vi "Main.vi"(8 "error in (no error)":errorcluster, 11 "GalvoBase in":refnum<class "ImagingModeSPIM.lvclass">) -> (0 "error out":errorcluster, 3 "component":refnum<class "ImagingModeSPIM.lvclass">)   [LabVIEW 2012, in "ImagingModeSPIM.lvclass"]
doc: "Main VI of the component."
uses:
  ImagingModeSPIM.lvclass
  Controls/wavelength_ring.ctl
  ImagingModeSPIM.lvclass/ImagingModeSPIM.ctl
  <vilib>/Distrio/Murmex/InitialiseMessage/InitialiseMessage.lvclass
  <vilib>/Distrio/Murmex/TerminateMessage/TerminateMessage.lvclass
  <vilib>/Distrio/Murmex/ConfigureMessage/ConfigureMessage.lvclass
  <vilib>/Distrio/Murmex/StopMessage/StopMessage.lvclass
  <vilib>/Distrio/Murmex/StartMessage/run mode enum.ctl
  <vilib>/Distrio/Murmex/StartMessage/StartMessage.lvclass
  <vilib>/Distrio/Murmex/Murmex/update_cluster.ctl
  <vilib>/Distrio/Murmex/Murmex/Set configure at initialise.vi
  <vilib>/Distrio/Murmex/Murmex/Set VI reference.vi
  <vilib>/Distrio/Murmex/Murmex/Get ID.vi
  <vilib>/Distrio/Murmex/Murmex/Set relay start stop to observers.vi
  <vilib>/Distrio/Murmex/Murmex/Set log reference.vi
  <vilib>/Distrio/Murmex/Murmex/Set license required.vi
  <vilib>/Distrio/Murmex/Murmex/Set write log to disk.vi
  <vilib>/Distrio/Murmex/StartMessage/Set run mode.vi
  <vilib>/Distrio/Murmex/Murmex/Murmex.lvclass
panel:
  in  "button::quit":bool
  in  "button:start_finite":bool
  in  "button:start_free-run":bool
  in  "button::configure":bool
  in  "Tab Control":T1(tab)
  in  "Phase 2":dbl[unit] caption="phase" min=-6.283185307179586 max=6.283185307179586 step=0.0017453292519943296
  in  "Offset 2":dbl[unit] caption="offset" min=-5.0 max=5.0 step=0.01
  in  "Amplitude 2":dbl[unit]=1.0 caption="amplitude" min=0.0 max=5.0 step=0.01
  in  "Phase 1":dbl[unit] caption="phase" min=-6.283185307179586 max=6.283185307179586 step=0.0017453292519943296
  in  "Offset 1":dbl[unit] caption="offset" min=-5.0 max=5.0 step=0.01
  in  "Amplitude 1":dbl[unit]=1.0 caption="amplitude" min=0.0 max=5.0 step=0.01
  out "Offset_slow":dbl[unit] caption="offset"
  out "step_size":dbl[unit]=1.0 caption="step size"
  in  "Phase_fast":dbl[unit]=3.141593 caption="phase" min=-6.283185307179586 max=6.283185307179586 step=0.0017453292519943296
  in  "Offset_fast":dbl[unit] caption="offset" min=-5.0 max=5.0 step=0.01
  in  "Amplitude_fast":dbl[unit]=0.5 caption="amplitude" min=-10.0 max=10.0 step=0.01
  out "write to task counter":i32
  out "data sent":dbl[unit]
  out "frequency slow":dbl[unit]
  in  "additional offset":dbl[unit]
  out "frame rate":dbl[unit]=100.0
  out "HSYNC pulses":i32=2048 min=4 max=2048 step=4
  in  "Wavelength":T2 items=["405nm"=0.14, "445nm"=0.34, "491nm"=0.41, "515nm"=0.17, "561nm"=0.5]
  in  "digital ratio":dbl(knob)=0.5 min=0.0 max=1.0 step=0.02 scale=0.0..1.0
  in  "pulses per pixel":i32=2 min=0 max=20 step=2
  out "log":string
  in  "ID":string="spim"
  out "terminate?":bool=TRUE
  # "galvo 1"
  # "galvo 2"
  # "fast scan"
  # "slow scan"
  # "Prato"
  # "Florence"
  # "ImagingModeSPIM\n\nDeveloped by:\n\nMarcel van 't Hoff PhD, \nMarie Caroline Muellenbroich PhD, \nLudovico Silvestri PhD,\nUniversity of Florence, 2014"
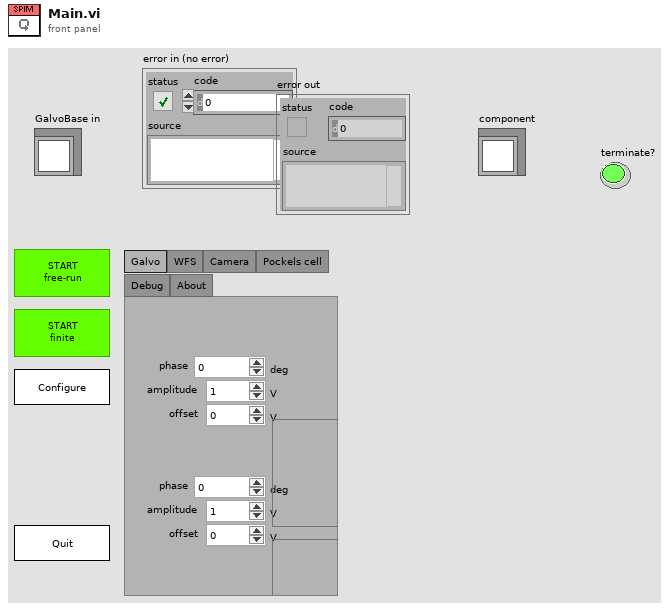
[diagram p1: front panel]
types:
  T1 = enum32{"Galvo", "WFS", "Camera", "Pockels cell", "Debug", "About"}
  T2 = typedef "ImagingModeSPIM.lvclass/wavelength_ring.ctl" = dbl
  T3 = enum8{"Enabled", "Disabled", "Disabled and Grayed Out"}
  T4 = typedef "Murmex.lvlib/StartMessage.lvclass/run mode enum.ctl" = enum16{"infinite", "finite"}
  T5 = typedef "Murmex.lvlib/Murmex.lvclass/update_cluster.ctl" = cluster{"target ID":string, "key chains":string[], "values":variant[]}
  T6 = typedef "Murmex.lvlib/Murmex.lvclass/command_enum.ctl" = enum16{"null", "initialise", "reset", "terminate", "acknowledge", "update", "inspect", "inform", "proceed", "start", "stop", "fetch", "configure", "generic"}
  T7 = typedef "Murmex.lvlib/Murmex.lvclass/Event type enumerations.ctl" = enum16{"before", "after"}
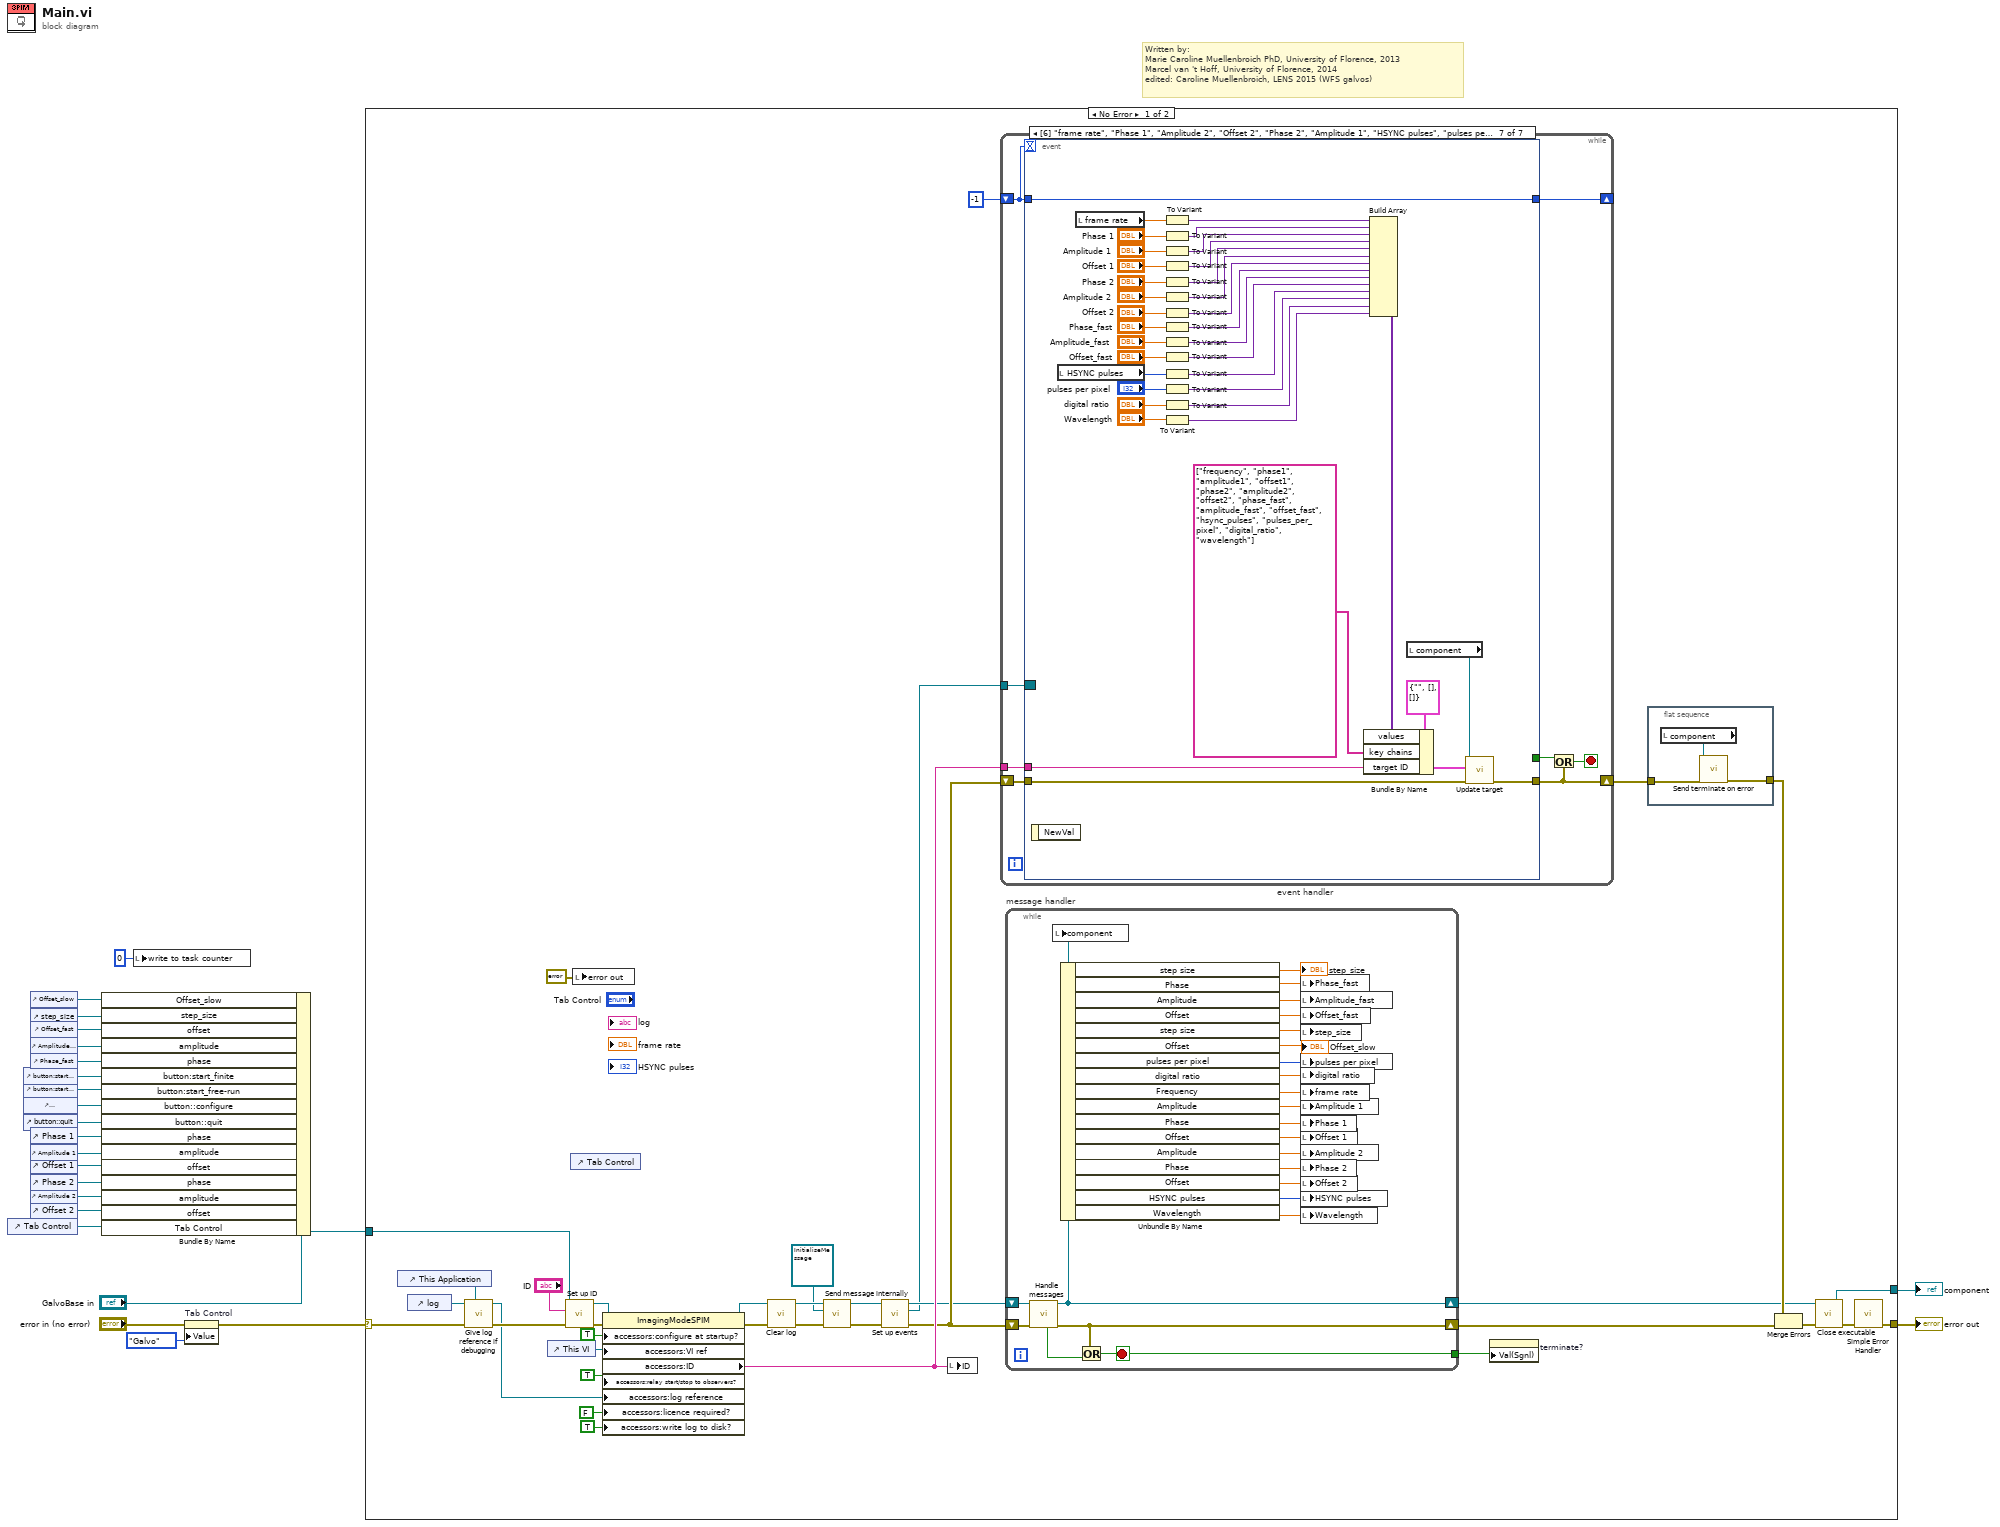
[diagram p0: block diagram]
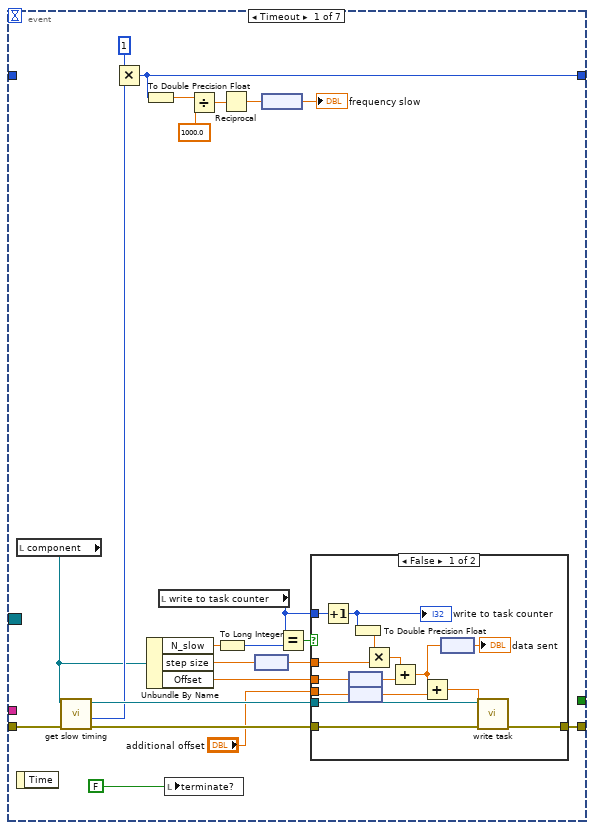
[diagram p2: hidden frame]
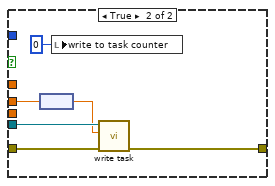
[diagram p3: hidden frame]
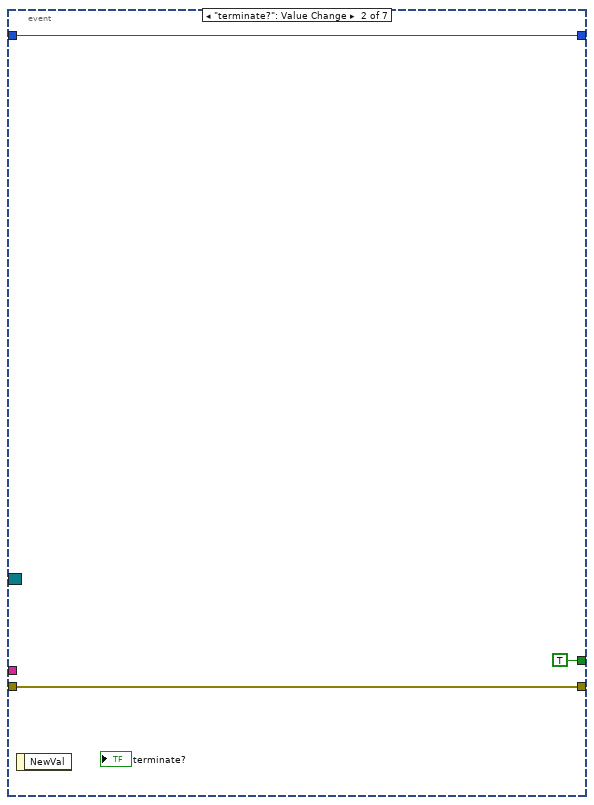
[diagram p4: hidden frame]
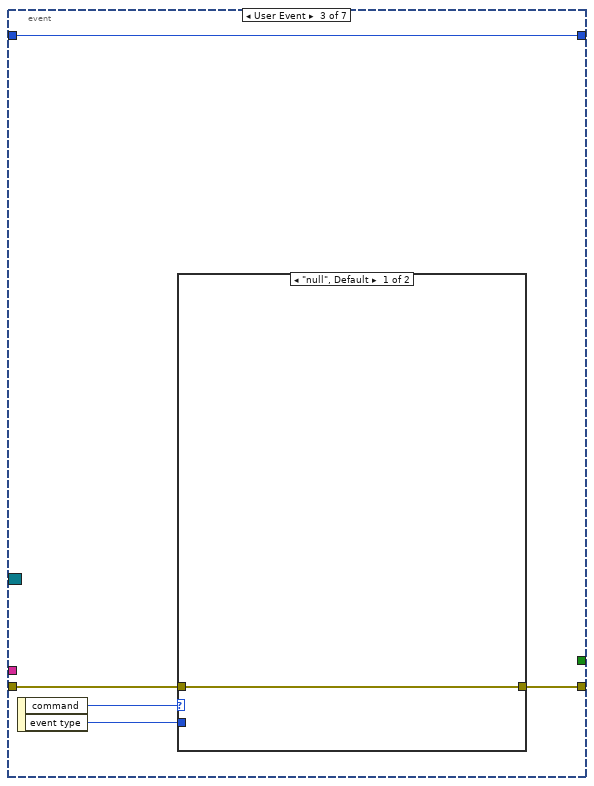
[diagram p5: hidden frame]
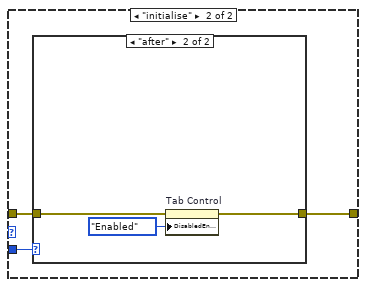
[diagram p6: hidden frame]
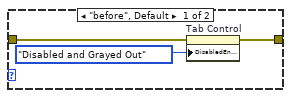
[diagram p7: hidden frame]
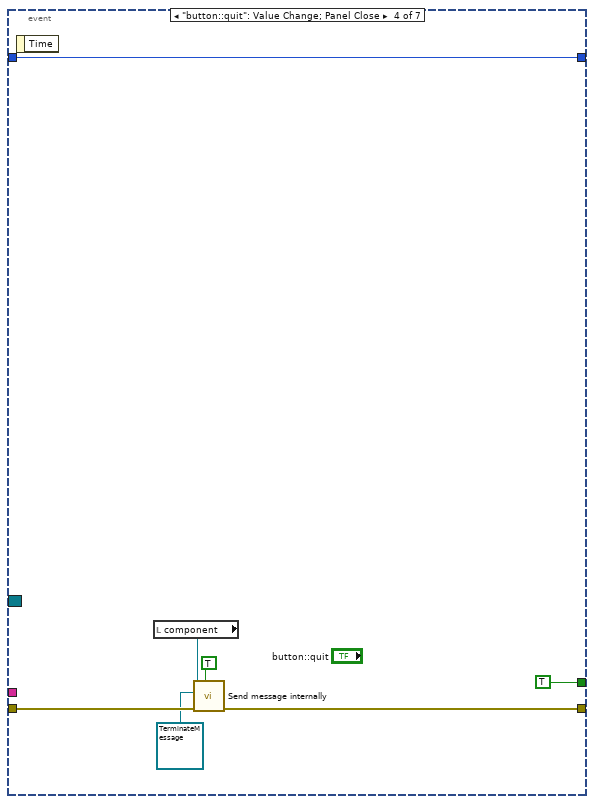
[diagram p8: hidden frame]
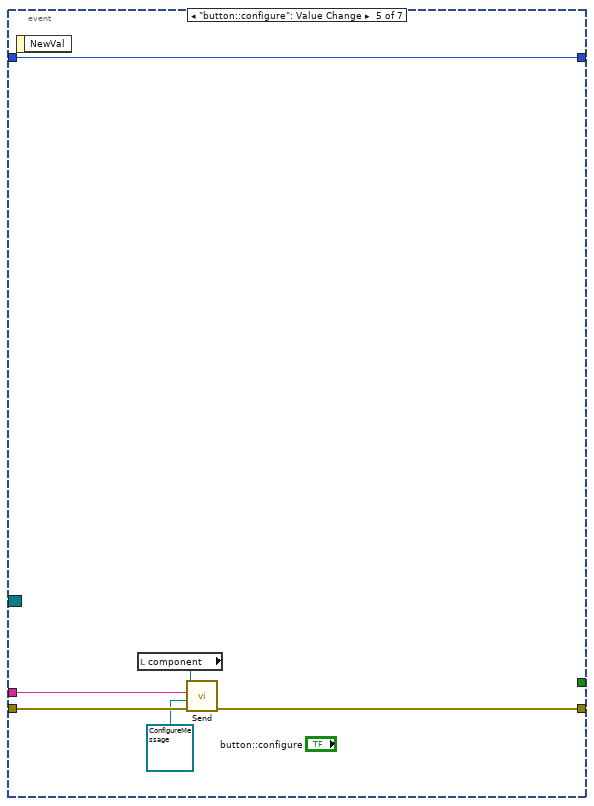
[diagram p9: hidden frame]
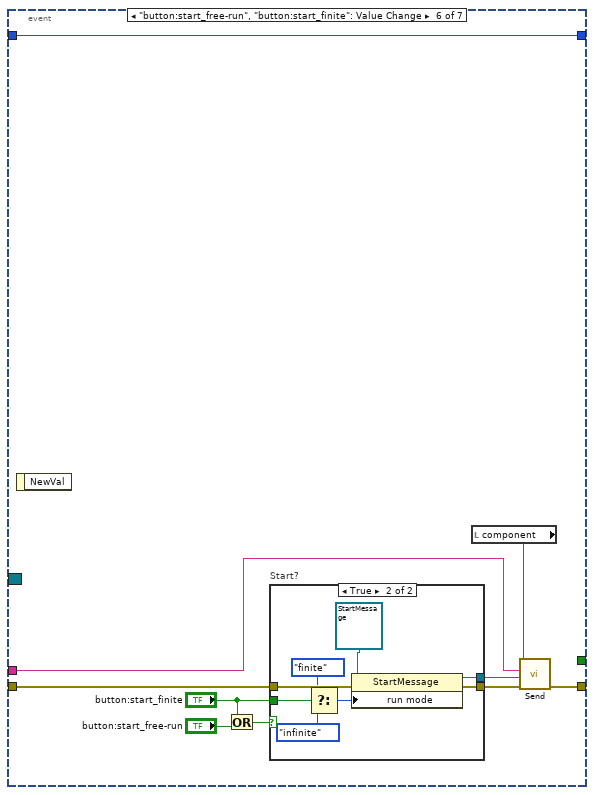
[diagram p10: hidden frame]
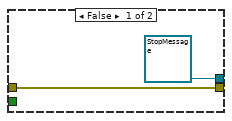
[diagram p11: hidden frame]
diagram:
  # "Written by:\nMarie Caroline Muellenbroich PhD, University of Florence, 2013 \nMarcel van 't Hoff, University of Florence, 2014\nedited: Caroline Muellenbroich, LENS 2015 (WFS galvos)"
  n1 = control-ref of="Tab Control"() -> (w4:refnum<vi>)
  n2 = control-ref of="button:start_finite"() -> (w21:refnum<vi>)
  n3 = control-ref of="button:start_free-run"() -> (w18:refnum<vi>)
  n4 = control-ref of="button::configure"() -> (w19:refnum<vi>)
  n5 = control-ref of="button::quit"() -> (w20:refnum<vi>)
  n6 = control-ref of="Offset_slow"() -> (w3:refnum<vi>)
  n7 = control-ref of="step_size"() -> (w2:refnum<vi>)
  n8 = control-ref of="Offset_fast"() -> (w6:refnum<vi>)
  n9 = control-ref of="Amplitude_fast"() -> (w7:refnum<vi>)
  n10 = control-ref of="Phase_fast"() -> (w8:refnum<vi>)
  n11 = control-ref of="Phase 1"() -> (w17:refnum<vi>)
  n12 = control-ref of="Amplitude 1"() -> (w16:refnum<vi>)
  n13 = control-ref of="Offset 1"() -> (w15:refnum<vi>)
  n14 = control-ref of="Phase 2"() -> (w14:refnum<vi>)
  n15 = control-ref of="Amplitude 2"() -> (w13:refnum<vi>)
  n16 = control-ref of="Offset 2"() -> (w12:refnum<vi>)
  n17 = Bundle By Name(cluster="GalvoBase in", "Offset_slow"=w3, "step_size"=w2, "offset"=w6, "amplitude"=w7, "phase"=w8, "button:start_finite"=w21, "button:start_free-run"=w18, "button::configure"=w19, "button::quit"=w20, "phase"=w17, "amplitude"=w16, "offset"=w15, "phase"=w14, "amplitude"=w13, "offset"=w12, "Tab Control"=w4) -> (w22:refnum<class "ImagingModeSPIM.lvclass">)
  n18 = local write "write to task counter"(0 ("write to task counter")) -> ()
  n19 = property on="Tab Control" class="TabCtl (strict)"(error in="error in (no error)", "Value"=T1."Galvo" ("Tab Control")) -> (error out=w9:errorcluster)  [unwired: 1 in, 1 out]
  n20 = case shown="No Error" w9 {
    selector: w9 -> [w30 w226]
    tunnel: [w60 w226] -> w24
    tunnel: w22 -> [w42 w227]
    tunnel: [w59 w227] -> w10
    frame No Error {
      n21 = control-ref of="This Application"() -> (w26:refnum<vi>)
      n22 = control-ref of="log"() -> (w28:refnum<vi>)
      n23 = call "Give log reference if debugging.vi"("application ref"=w26, "error in (no error)"=w30, "log reference in"=w28) -> ("error out"=w29:errorcluster, "log reference out"=w27:refnum<vi>)  [unwired: 6 in, 1 out]
      n24 = control-ref of="This VI"() -> (w57:refnum<vi>)
      n25 = call <vilib>:"Set up ID.vi"("error in (no error)"=w29, "component ID"="ID", "MurmexBase in"=w42) -> ("error out"=w54:errorcluster, "MurmexBase out"=w55:refnum<class "ImagingModeSPIM.lvclass">)  [unwired: 6 in, 1 out]
      n26 = control-ref of="Tab Control"() -> ()  [unwired: 1 out]
      n27 = local write "error out"(errorcluster {"status"=FALSE, "code"=0, "source"=""} ("error out")) -> ()
      n28 = property class="ImagingModeSPIM"(reference=w55, error in=w54, "accessors:configure at startup?"=TRUE ("configure at startup?"), "accessors:VI ref"=w57, "accessors:relay start/stop to observers?"=TRUE ("relay start/stop to observers?"), "accessors:log reference"=w27, "accessors:licence required?"=FALSE ("licence required?"), "accessors:write log to disk?"=TRUE ("write log to disk?")) -> (reference out=w39:refnum<class "ImagingModeSPIM.lvclass">, error out=w41:errorcluster, "accessors:ID"=w44:string)
      n29 = call <vilib>:"Clear log.vi"("error in (no error)"=w41, "MurmexBase in"=w39) -> ("error out"=w40:errorcluster, "MurmexBase out"=w38:refnum<class "ImagingModeSPIM.lvclass">)  [unwired: 8 in]
      n30 = call <vilib>:"Send message internally.vi"("error in (no error)"=w40, "Message"=refnum<class "InitialiseMessage.lvclass"> refnum ("Murmex.lvlib:InitialiseMessage"), "Murmex in"=w38) -> ("error out"=w35:errorcluster, "Murmex out"=w33:refnum<class "ImagingModeSPIM.lvclass">)  [unwired: 7 in]
      n31 = call <vilib>:"Set up events.vi"("error in (no error)"=w35, "MurmexBase in"=w33) -> ("error out"=w34:errorcluster, "Event Registration Refnum"=w31:refnum<event-registration>, "MurmexBase out"=w32:refnum<class "ImagingModeSPIM.lvclass">)  [unwired: 7 in]
      n32 = local write "ID"(w44) -> ()
      n33 = while "event handler" {
        shift-right: [w69] -> w52
        shift-left: w34 -> [w71]
        shift-right: [w65] -> _
        shift-left: -1 -> [w66]
        tunnel: w44 -> [w67]
        tunnel: w31 -> [w64]
        stop <- w68 stop-if-true
        n34 = event shown="[6] \"frame rate\", \"Phase 1\", \"Amplitude 2\", \"Offset 2\", \"Phase 2\", \"Amplitude 1\", \"HSYNC pulses\", \"pulses per pixel\", \"digital ratio\", \"Wavelength\", \"Offset_slow\", \"step_size\", \"Phase_fast\", \"Offset_fast\", \"Amplitude_fast\", \"Offset 1\": Value Change" {
          selector: w64 -> [_ _ _ _ _ _ _]
          dyn-events: _ -> [_ _ _ _ _ _ _]
          timeout: w66 -> [_ _ _ _ _ _ _]
          tunnel: [w92 w117 w119 w139 w144 w149 w201] -> w69
          tunnel: w71 -> [w91 w117 w120 w138 w145 w154 w202]
          tunnel: [_ TRUE ("configure at startup?") _ TRUE ("configure at startup?") _ _ _] -> w70
          tunnel: w67 -> [_ _ _ _ w143 w146 w183]
          tunnel: w66 -> [_ w115 w118 w136 w142 w155 w189]
          tunnel: [w78 w115 w118 w136 w142 w155 w189] -> w65
          event Timeout {
            n35 = local read "component"() -> (w86:refnum<class "ImagingModeSPIM.lvclass">)
            n36 = event-data() -> ()  [unwired: 1 in, 1 out]
            n37 = call-dynamic "get slow timing.vi"("error in (no error)"=w91, "ImagingModeSPIM in"=w86) -> ("error out"=w90:errorcluster, "frame rate"=w87:i32, "ImagingModeSPIM out"=w89:refnum<class "ImagingModeSPIM.lvclass">)  [unwired: 6 in, 1 out]
            n38 = Multiply(x=1, y=w87) -> (x*y=w78:i32)
            n39 = To Double Precision Float(number=w78) -> (double precision float=w77:dbl)
            n40 = Unbundle By Name(w86) -> ("N_slow"=w85:dbl, "step size"=w74:dbl[unit], "Offset"=w80:dbl[unit])
            n41 = local read "write to task counter"() -> (w83:i32)
            n42 = local write "terminate?"(FALSE ("terminate?")) -> ()
            n43 = Divide(x=w77, y=1000.0) -> (x/y=w76:dbl)
            n44 = To Long Integer(number=w85) -> (32bit integer=w82:i32)
            n45 = Reciprocal(x=w76) -> (1/x=w75:dbl)
            n46 = node(w74) -> (w81:dbl)
            n47 = node(w75) -> (→"frequency slow":dbl[unit])
            n48 = Equal?(x=w83, y=w82) -> (x = y?=w84:bool)
            n49 = case shown="False" w84 {
              tunnel: [w107 w114] -> w92
              tunnel: w90 -> [w108 w113]
              tunnel: w89 -> [w106 w112]
              tunnel: w83 -> [w105 _]
              tunnel: w81 -> [w103 _]
              tunnel: w80 -> [w100 w109]
              tunnel: "additional offset" -> [w95 _]
              frame False {
                n50 = Increment(x=w105) -> (x+1=w102:i32)
                "write to task counter" <- w102
                n51 = node(w100) -> (w99:dbl)
                n52 = node(w95) -> (w94:dbl)
                n53 = To Double Precision Float(number=w102) -> (double precision float=w104:dbl)
                n54 = Multiply(x=w104, y=w103) -> (x*y=w101:dbl)
                n55 = Add(x=w101, y=w99) -> (x+y=w98:dbl)
                n56 = Add(x=w98, y=w94) -> (x+y=w96:dbl)
                n57 = node(w98) -> (→"data sent":dbl[unit])
                n58 = call-dynamic "write task.vi"("error in (no error)"=w108, "data"=w96, "ImagingModeSPIM in"=w106) -> ("error out"=w107:errorcluster)  [unwired: 7 in, 1 out]
              }
              frame True {
                n59 = node(w109) -> (w110:dbl)
                n60 = local write "write to task counter"(0 ("write to task counter")) -> ()
                n61 = call-dynamic "write task.vi"("error in (no error)"=w113, "data"=w110, "ImagingModeSPIM in"=w112) -> ("error out"=w114:errorcluster)  [unwired: 7 in, 1 out]
              }
            }
          }
          event "terminate?": Value Change {
            n62 = event-data() -> ()  [unwired: 1 in, 1 out]
          }
          event User Event {
            n63 = event-data() -> ("command"=w122:T6, "event type"=w121:T7)  [unwired: 1 in]
            n64 = case shown="\"null\", Default" w122 {
              tunnel: w121 -> [_ w126]
              tunnel: w120 -> [w123 w125]
              tunnel: [w123 w124] -> w119
              frame "null", Default {
              }
              frame "initialise" {
                n65 = case shown="\"after\"" w126 {
                  tunnel: w125 -> [w129 w132]
                  tunnel: [w128 w131] -> w124
                  frame "before", Default {
                    n66 = property on="Tab Control" class="TabCtl (strict)"(error in=w129, "DisabledEnum"=T3."Disabled and Grayed Out" ("Disabled")) -> (error out=w128:errorcluster)  [unwired: 1 in, 1 out]
                  }
                  frame "after" {
                    n67 = property on="Tab Control" class="TabCtl (strict)"(error in=w132, "DisabledEnum"=T3."Enabled" ("Disabled")) -> (error out=w131:errorcluster)  [unwired: 1 in, 1 out]
                  }
                }
              }
            }
          }
          event "button::quit": Value Change; Panel Close {
            n68 = event-data() -> ()  [unwired: 1 in, 1 out]
            n69 = local read "component"() -> (w135:refnum<class "ImagingModeSPIM.lvclass">)
            n70 = call <vilib>:"Send message internally.vi"("priority message? (F)"=TRUE, "error in (no error)"=w138, "Message"=refnum<class "TerminateMessage.lvclass"> refnum ("Murmex.lvlib:TerminateMessage"), "Murmex in"=w135) -> ("error out"=w139:errorcluster)  [unwired: 6 in, 1 out]
          }
          event "button::configure": Value Change {
            n71 = event-data() -> ()  [unwired: 1 in, 1 out]
            n72 = local read "component"() -> (w141:refnum<class "ImagingModeSPIM.lvclass">)
            n73 = call <vilib>:"Send.vi"("error in (no error)"=w145, "Message"=refnum<class "ConfigureMessage.lvclass"> refnum ("Murmex.lvlib:ConfigureMessage"), "recipient"=w143, "Murmex in"=w141) -> ("error out"=w144:errorcluster)  [unwired: 6 in, 1 out]
          }
          event "button:start_free-run", "button:start_finite": Value Change {
            n74 = event-data() -> ()  [unwired: 1 in, 1 out]
            n75 = Or(x="button:start_finite", y="button:start_free-run") -> (x .or. y?=w153:bool)
            n76 = case "Start?" shown="True" w153 {
              tunnel: w154 -> [w157 w165]
              tunnel: [w157 w160] -> w150
              tunnel: "button:start_finite" -> [_ w161]
              tunnel: [refnum<class "StopMessage.lvclass"> refnum ("Murmex.lvlib:StopMessage") w159] -> w147
              frame False {
              }
              frame True {
                n77 = Select(t=run_mode_enum."finite" ("run mode"), s=w161, f=run_mode_enum."infinite" ("run mode")) -> (s? t:f=w162:T4)
                n78 = property class="StartMessage"(reference=refnum<class "StartMessage.lvclass"> refnum ("Murmex.lvlib:StartMessage"), error in=w165, "run mode"=w162) -> (reference out=w159:refnum<class "StartMessage.lvclass">, error out=w160:errorcluster)
              }
            }
            n79 = local read "component"() -> (w148:refnum<class "ImagingModeSPIM.lvclass">)
            n80 = call <vilib>:"Send.vi"("error in (no error)"=w150, "Message"=w147, "recipient"=w146, "Murmex in"=w148) -> ("error out"=w149:errorcluster)  [unwired: 6 in, 1 out]
          }
          event "frame rate", "Phase 1", "Amplitude 2", "Offset 2", "Phase 2", "Amplitude 1", "HSYNC pulses", "pulses per pixel", "digital ratio", "Offset_slow", "step_size", "Phase_fast", "Offset_fast", "Amplitude_fast", "Offset 1": Value Change {
            n81 = event-data() -> ()  [unwired: 1 in, 1 out]
            n82 = local read "HSYNC pulses"() -> (w180:i32)
            n83 = local read "frame rate"() -> (w179:dbl[unit])
            n84 = To Variant(anything=w179) -> (Variant=w198:variant)
            n85 = To Variant(anything="Phase 1") -> (Variant=w195:variant)
            n86 = To Variant(anything="Amplitude 1") -> (Variant=w194:variant)
            n87 = To Variant(anything="Offset 1") -> (Variant=w193:variant)
            n88 = To Variant(anything="Phase 2") -> (Variant=w187:variant)
            n89 = To Variant(anything="Amplitude 2") -> (Variant=w186:variant)
            n90 = To Variant(anything="Offset 2") -> (Variant=w184:variant)
            n91 = To Variant(anything="Phase_fast") -> (Variant=w173:variant)
            n92 = To Variant(anything="Amplitude_fast") -> (Variant=w172:variant)
            n93 = To Variant(anything="Offset_fast") -> (Variant=w171:variant)
            n94 = To Variant(anything=w180) -> (Variant=w170:variant)
            n95 = To Variant(anything="pulses per pixel") -> (Variant=w169:variant)
            n96 = To Variant(anything="digital ratio") -> (Variant=w168:variant)
            n97 = To Variant(anything="Wavelength") -> (Variant=w167:variant)
            n98 = Build Array(w198, w195, w194, w193, w187, w186, w184, w173, w172, w171, w170, w169, w168, w167) -> (w197:variant[])
            n99 = Bundle By Name(cluster=T5 {"target ID"="", "key chains"=[], "values"=[]} ("update cluster"), "values"=w197, "key chains"=string[] ["frequency", "phase1", "amplitude1", "offset1", "phase2", "amplitude2", "offset2", "phase_fast", "amplitude_fast", "offset_fast", "hsync_pulses", "pulses_per_pixel", "digital_ratio", "wavelength"], "target ID"=w183) -> (w199:T5)
            n100 = local read "component"() -> (w178:refnum<class "ImagingModeSPIM.lvclass">)
            n101 = call <vilib>:"Update target.vi"("error in (no error)"=w202, "update cluster"=w199, "MurmexBase in"=w178) -> ("error out"=w201:errorcluster)  [unwired: 7 in, 1 out]
          }
        }
        n102 = Or(x=w70, y=w69) -> (x .or. y?=w68:bool)
      }
      n103 = while "message handler" {
        shift-right: [w218] -> w47
        shift-left: w32 -> [w224]
        shift-right: [w205] -> w50
        shift-left: w34 -> [w225]
        tunnel: [w222] -> w56
        stop <- w222 stop-if-true
        n104 = call <vilib>:"Handle messages.vi"("error in (no error)"=w225, "Murmex in"=w224) -> ("error out"=w205:errorcluster, "Murmex out"=w218:refnum<class "ImagingModeSPIM.lvclass">, "terminated?"=w223:bool)  [unwired: 7 in]
        n105 = local write "component"(w218) -> ()
        n106 = Unbundle By Name(w218) -> ("step size"=→"step_size":dbl[unit], "Phase"=w206:dbl[unit], "Amplitude"=w207:dbl[unit], "Offset"=w208:dbl[unit], "step size"=w209:dbl[unit], "Offset"=→"Offset_slow":dbl[unit], "pulses per pixel"=w219:i32, "digital ratio"=w220:dbl, "Frequency"=w217:dbl[unit], "Amplitude"=w210:dbl[unit], "Phase"=w211:dbl[unit], "Offset"=w212:dbl[unit], "Amplitude"=w213:dbl[unit], "Phase"=w214:dbl[unit], "Offset"=w215:dbl[unit], "HSYNC pulses"=w221:i32, "Wavelength"=w216:T2)
        n107 = Or(x=w205, y=w223) -> (x .or. y?=w222:bool)
        n108 = local write "Phase_fast"(w206) -> ()
        n109 = local write "Amplitude_fast"(w207) -> ()
        n110 = local write "Offset_fast"(w208) -> ()
        n111 = local write "step_size"(w209) -> ()
        n112 = local write "pulses per pixel"(w219) -> ()
        n113 = local write "digital ratio"(w220) -> ()
        n114 = local write "frame rate"(w217) -> ()
        n115 = local write "Amplitude 1"(w210) -> ()
        n116 = local write "Phase 1"(w211) -> ()
        n117 = local write "Offset 1"(w212) -> ()
        n118 = local write "Amplitude 2"(w213) -> ()
        n119 = local write "Phase 2"(w214) -> ()
        n120 = local write "Offset 2"(w215) -> ()
        n121 = local write "HSYNC pulses"(w221) -> ()
        n122 = local write "Wavelength"(w216) -> ()
      }
      n123 = property on="terminate?" class="Bool (strict)"("Val(Sgnl)"=w56) -> ()  [unwired: 2 in, 2 out]
      n124 = flat-sequence {
        tunnel: w52 -> [w63]
        tunnel: [w61] -> w51
        frame #0 {
          n125 = local read "component"() -> (w62:refnum<class "ImagingModeSPIM.lvclass">)
          n126 = call <vilib>:"Send terminate on error.vi"("error in (no error)"=w63, "Murmex in"=w62) -> ("error out"=w61:errorcluster)  [unwired: 8 in, 1 out]
        }
      }
      n127 = Merge Errors(w51, w50) -> (w49:errorcluster)
      n128 = call <vilib>:"Close executable.vi"("error in (no error)"=w49, "MurmexBase in"=w47) -> ("error out"=w48:errorcluster, "MurmexBase out"=w59:refnum<class "ImagingModeSPIM.lvclass">)  [unwired: 8 in]
      n129 = call <vilib>:"Simple Error Handler.vi"("error in (no error)"=w48) -> ("error out"=w60:errorcluster)  [unwired: 4 in, 4 out]
    }
    frame Error {
    }
  }
  "error out" <- w24
  "component" <- w10
